vi "configureUnique.vi"(8 "error in (no error)":errorcluster, 10 "Data":u8[](array[numeric]), 11 "Mockbus in":refnum<class "Mockbus.lvclass">) -> (0 "error out":errorcluster, 3 "Mockbus out":refnum<class "Mockbus.lvclass">)   [LabVIEW 2015, in "RTMockbus.lvlib" / "Mockbus.lvclass"]
uses:
  Mockbus.lvclass
  Mockbus.lvclass/Mockbus.ctl
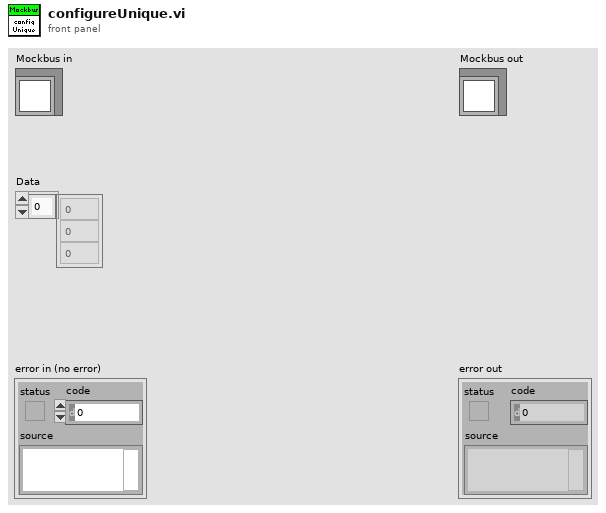
[diagram p1: front panel]
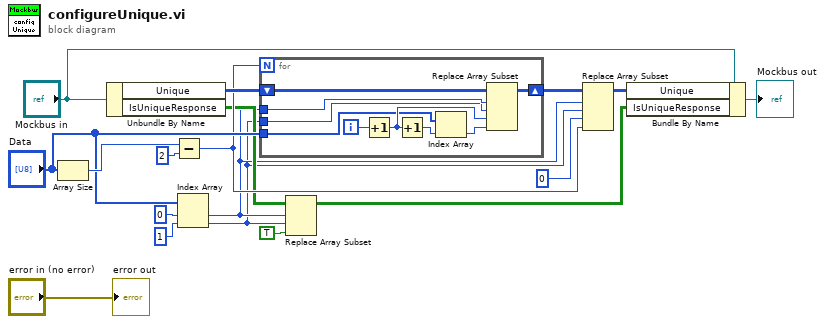
[diagram p0: block diagram]
diagram:
  n1 = Array Size(array="Data") -> (size(s)=w13:i32)
  n2 = Unbundle By Name("Mockbus in") -> ("Unique"=w10:u8[][][], "IsUniqueResponse"=w5:bool[][])
  n3 = Subtract(x=w13, y=2) -> (x-y=w7:i32)
  n4 = Index Array(array="Data", index #1=0 ("index"), index #2=1 ("index")) -> (element #1=w4:u8, element #2=w3:u8)
  n5 = for {
    N: w7 -> [_]
    tunnel: "Data" -> [w19]
    tunnel: w4 -> [w26]
    tunnel: w3 -> [w25]
    shift-right: [w24] -> w9
    shift-left: w10 -> [w27]
    i -> [w22]
    n6 = Increment(x=w22) -> (x+1=w23:i32)
    n7 = Increment(x=w23) -> (x+1=w21:i32)
    n8 = Index Array(array=w19, index=w21) -> (element=w20:u8)
    n9 = Replace Array Subset(array=w27, new element=w20, index (dim 0)=w26, index (dim 1)=w25, index (dim 2)=w23) -> (w24:u8[][][])
  }
  n10 = Replace Array Subset(array=w5, new element=TRUE ("new element/subarray"), index (row)=w4, index (col)=w3) -> (w1:bool[][])
  n11 = Replace Array Subset(array=w9, new element=w7, index (dim 0)=w4, index (dim 1)=w3, index (dim 2)=0 ("disabled index (col)")) -> (w6:u8[][][])
  n12 = Bundle By Name(cluster="Mockbus in", "Unique"=w6, "IsUniqueResponse"=w1) -> (→"Mockbus out":refnum<class "Mockbus.lvclass">)
  "error out" <- "error in (no error)"
